vi "USB2XXX_PWM_SnifferTest.vi"() -> ()   [LabVIEW 2010]
panel:
  in  "TimePrecUs":u8=10
  out "占空比":dbl
  out "频率":dbl
  in  "pPWMData":cluster{"LowValue":u16, "HighValue":u16}
  out "pPWMData out":cluster{"LowValue":u16, "HighValue":u16}
  in  "stop":bool
  in  "Channel":u8
  in  "Device Index":i32(ring) items=["0", "1", "2", "3", "4", "5"]
  # "通道0-->LIN1-->P1"
  # "通道1-->LIN2-->P6"
  # "KHz"
  # "%"
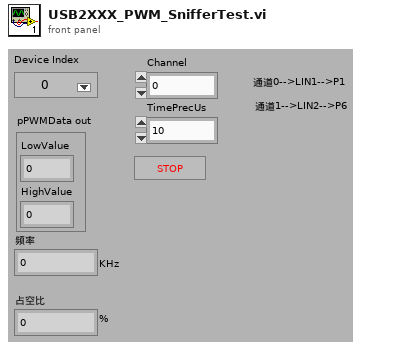
[diagram p1: front panel]
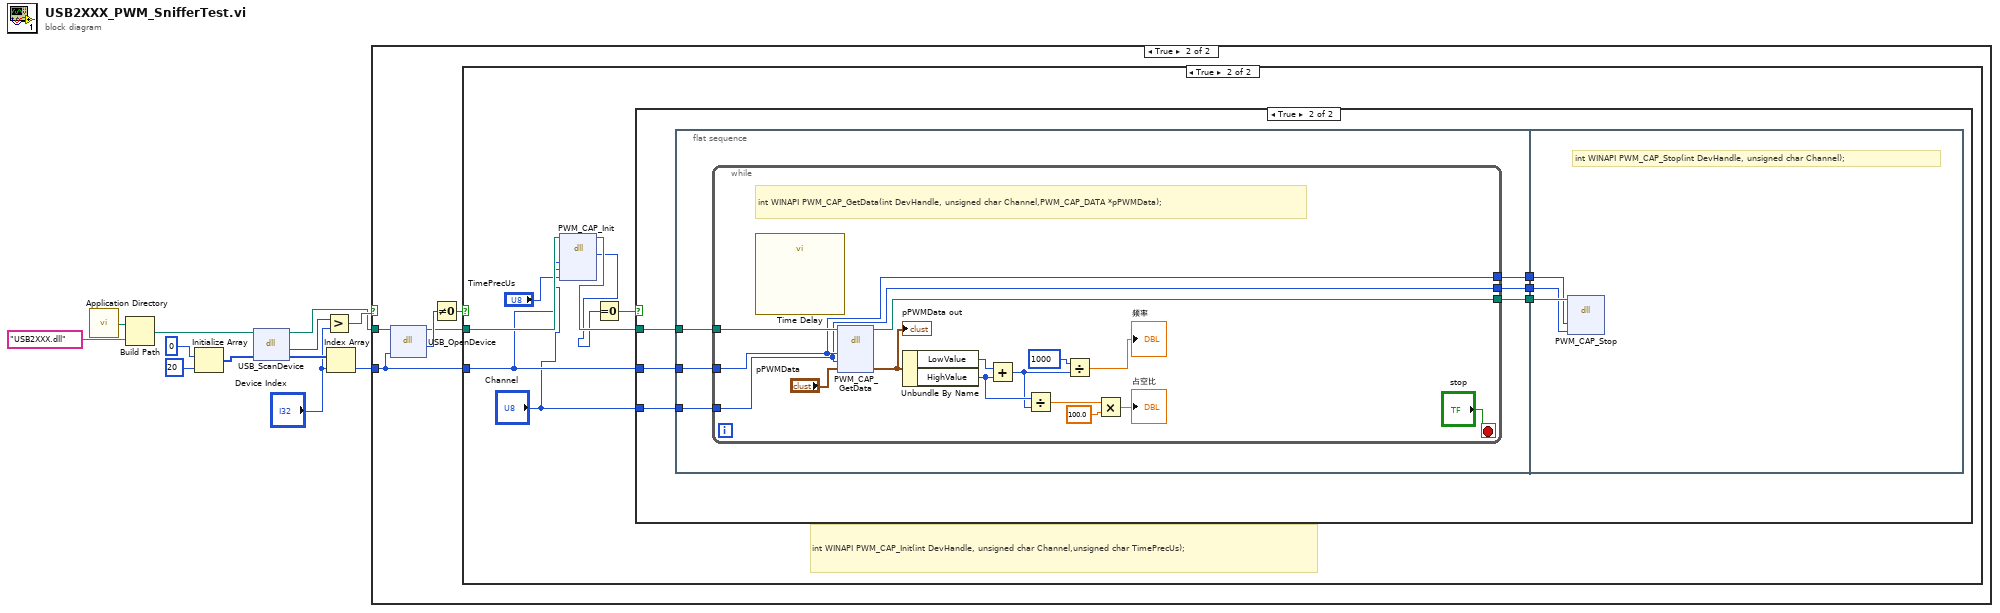
[diagram p0: block diagram]
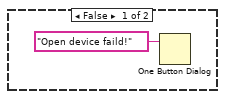
[diagram p3: hidden frame]
diagram:
  n1 = call <vilib>:"Application Directory.vi"() -> ("Application Directory"=w3:path)
  n2 = Build Path(base path=w3, name or relative path="USB2XXX.dll") -> (appended path=w2:path)
  n3 = Initialize Array(0, 20 ("dimension size")) -> (w9:i32[])
  n4 = dll-call lib="E:/Projects/USB2XXX_Example/sdk/api/Labview/USB2XXX.*" fn="USB_ScanDevice"(path in=w2, "pDevNum"=w9) -> (path out=w1:path, "return type"=w8:i32, "pDevNum"=w12:i32[])  [unwired: 2 in, 1 out]
  n5 = Greater?(x=w8, y="Device Index") -> (0:w6:bool)
  n6 = Index Array(array=w12, index="Device Index") -> (element=w5:i32)
  n7 = case shown="True" w6 {
    tunnel: w5 -> [_ w15]
    tunnel: w1 -> [_ w14]
    frame False {
    }
    frame True {
      n8 = dll-call lib="E:/Projects/USB2XXX_Example/sdk/api/Labview/USB2XXX.*" fn="USB_OpenDevice"(path in=w14, "DevIndex"=w15) -> (path out=w13:path, "return type"=w17:u8)  [unwired: 3 in, 1 out]
      n9 = Not Equal To 0?(x=w17) -> (x != 0?=w16:bool)
      n10 = case shown="True" w16 {
        tunnel: w15 -> [_ w21]
        tunnel: w13 -> [_ w24]
        frame False {
          n11 = One Button Dialog(message="Open device faild!") -> ()  [unwired: 1 in, 1 out]
        }
        frame True {
          # "int WINAPI PWM_CAP_Init(int DevHandle, unsigned char Channel,unsigned char TimePrecUs);"
          n12 = dll-call lib="E:/Projects/USB2XXX/trunk/USB2XXX/USB2XXX/vs2010/Release/USB2XXX.*" fn="PWM_CAP_Init"(path in=w24, "DevHandle"=w21, "Channel"="Channel", "TimePrecUs"="TimePrecUs") -> (path out=w23:path, "return type"=w22:i32)  [unwired: 5 in, 1 out]
          n13 = Equal To 0?(x=w22) -> (x = 0?=w25:bool)
          n14 = case shown="True" w25 {
            tunnel: w21 -> [_ w31]
            tunnel: "Channel" -> [_ w30]
            tunnel: w23 -> [_ w29]
            frame False {
            }
            frame True {
              n15 = flat-sequence {
                tunnel: w31 -> [w37]
                tunnel: w30 -> [w36]
                tunnel: w29 -> [w35]
                tunnel: [w34] -> w28
                tunnel: [w33] -> w27
                tunnel: [w32] -> w26
                tunnel: w28 -> [w55]
                tunnel: w27 -> [w54]
                tunnel: w26 -> [w53]
                frame #0 {
                  n16 = while {
                    tunnel: w37 -> [w48]
                    tunnel: w36 -> [w47]
                    tunnel: w35 -> [w50]
                    tunnel: [w49] -> w34
                    tunnel: [w48] -> w33
                    tunnel: [w47] -> w32
                    stop <- "stop" stop-if-true
                    # "int WINAPI PWM_CAP_GetData(int DevHandle, unsigned char Channel,PWM_CAP_DATA *pPWMData);"
                    n17 = call "Time Delay"() -> ()  [unwired: 11 in, 1 out]
                    n18 = dll-call lib="E:/Projects/USB2XXX_Example/sdk/api/Labview/USB2XXX.*" fn="PWM_CAP_GetData"(path in=w50, "DevHandle"=w48, "Channel"=w47, "pPWMData"="pPWMData") -> (path out=w49:path, "pPWMData"=w46:cluster{"LowValue":u16, "HighValue":u16})  [unwired: 5 in, 1 out]
                    "pPWMData out" <- w46
                    n19 = Unbundle By Name(w46) -> ("LowValue"=w45:u16, "HighValue"=w42:u16)
                    n20 = Add(x=w45, y=w42) -> (x+y=w41:u16)
                    n21 = Divide(x=w42, y=w41) -> (x/y=w40:dbl)
                    n22 = Divide(x=u16 1000, y=w41) -> (x/y=→"频率":dbl)
                    n23 = Multiply(x=w40, y=100.0) -> (x*y=→"占空比":dbl)
                  }
                }
                frame #1 {
                  # "int WINAPI PWM_CAP_Stop(int DevHandle, unsigned char Channel);"
                  n24 = dll-call lib="E:/Projects/USB2XXX_Example/sdk/api/Labview/USB2XXX.*" fn="PWM_CAP_Stop"(path in=w55, "DevHandle"=w54, "Channel"=w53) -> ()  [unwired: 5 in, 2 out]
                }
              }
            }
          }
        }
      }
    }
  }
